vi "Teardown.vi"(11 "Event Transport in":refnum<class "Event Transport.lvclass">) -> (2 "Unhandled Msgs":refnum<class "Msg.lvclass">[](array[class]))   [LabVIEW 2025, in "jettl.lvlib" / "Transport.lvlib" / "Event.lvlib" / "Event Transport.lvclass"]
uses:
  Event Transport.lvclass
  Msg/Msg.lvclass
  Event Transport.lvclass/Event Transport.ctl
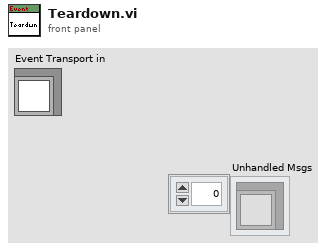
[diagram p1: front panel]
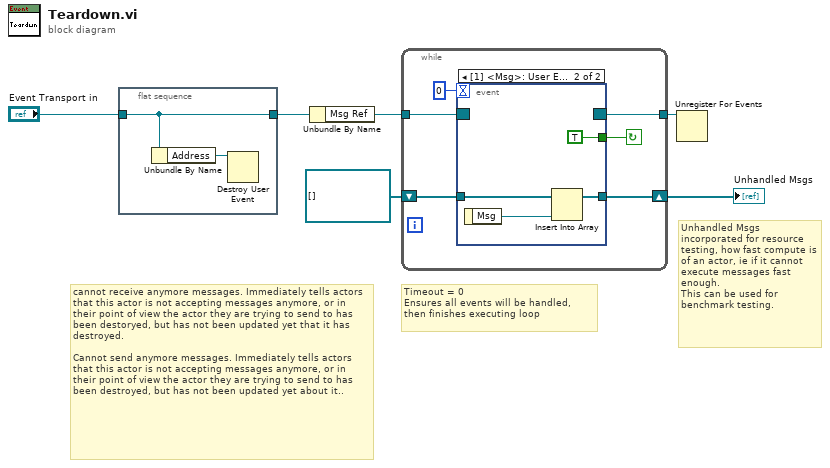
[diagram p0: block diagram]
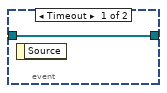
[diagram p2: hidden frame]
diagram:
  # "Unhandled Msgs incorporated for resource testing, how fast compute is of an actor, ie if it cannot execute messages fast enough.\nThis can be used for benchmark testing."
  # "Timeout = 0\nEnsures all events will be handled, then finishes executing loop"
  # "cannot receive anymore messages. Immediately tells actors that this actor is not accepting messages anymore, or in their point of view the actor they are trying to send to has been destoryed, but has not been updated yet that it has destroyed.\n\nCannot send anymore messages. Immediately tells actors that this actor is not accepting messages anymore, or in their point of view the actor they are trying to send to has been destroyed, but has not been updated yet about it.."
  n1 = flat-sequence {
    tunnel: "Event Transport in" -> [w8]
    tunnel: [w8] -> w2
    frame #0 {
      n2 = Unbundle By Name(w8) -> ("Address"=w7:refnum<user-event>)
      n3 = Destroy User Event(user event=w7) -> ()  [unwired: 1 in, 1 out]
    }
  }
  n4 = Unbundle By Name(w2) -> ("Msg Ref"=w1:refnum<event-registration>)
  n5 = while {
    shift-right: [w13] -> w4
    shift-left: refnum<class "Msg.lvclass">[] [] -> [w14]
    tunnel: w1 -> [w12]
    tunnel: [w9] -> w5
    stop <- w11 continue-if-true
    n6 = event shown="[1] <Msg>: User Event" {
      selector: w12 -> [_ _]
      dyn-events: [_ _] -> w9
      timeout: 0 -> [_ _]
      tunnel: w14 -> [w15 w19]
      tunnel: [w15 w18] -> w13
      tunnel: [_ TRUE] -> w11
      event Timeout {
        n7 = event-data() -> ()  [unwired: 1 in, 1 out]
      }
      event User Event {
        n8 = event-data() -> ("Msg"=w17:refnum<class "Msg.lvclass">)  [unwired: 1 in]
        n9 = Insert Into Array(array=w19, new element=w17) -> (w18:refnum<class "Msg.lvclass">[])  [unwired: 1 in]
      }
    }
  }
  "Unhandled Msgs" <- w4
  n10 = Unregister For Events(event registration refnum=w5) -> ()  [unwired: 1 in, 1 out]
